vi "Scan For App Projects.vi"(8 "error in":errorcluster, 10 "Init?":bool, 11 "Projects Ref":refnum<vi>) -> (0 "error out":errorcluster)   [LabVIEW 2019, in "Panther Dashboard.lvlib"]
uses:
  Panther Dashboard.lvlib
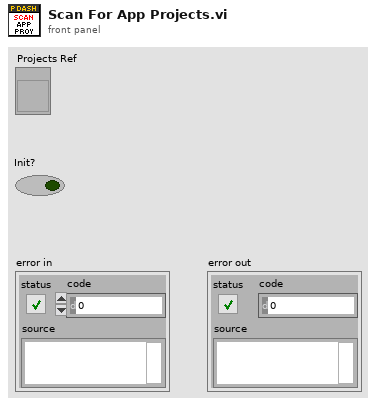
[diagram p1: front panel]
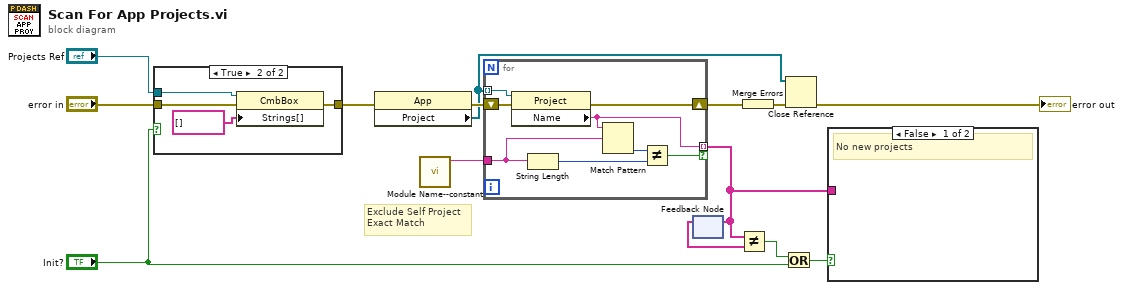
[diagram p0: block diagram]
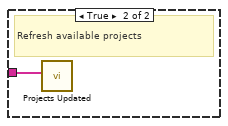
[diagram p3: hidden frame]
diagram:
  # "Exclude Self Project\nExact Match"
  n1 = case shown="True" "Init?" {
    tunnel: "Projects Ref" -> [_ w17]
    tunnel: "error in" -> [w15 w19]
    tunnel: [w15 w18] -> w11
    frame False {
    }
    frame True {
      n2 = property class="CmbBox"(reference=w17, error in=w19, "Strings[]"=string[] []) -> (error out=w18:errorcluster)  [unwired: 1 out]
    }
  }
  n3 = property class="App"(error in=w11) -> (error out=w9:errorcluster, "Project"=w8:refnum<vi>[])  [unwired: 1 in, 1 out]
  n4 = call "Module Name--constant.vi"() -> ("Module Name"=w1:string)  [unwired: 11 in]
  n5 = for {
    tunnel: w8 -> [w22] mode=indexing
    tunnel: [w25] -> w6 mode=indexing if=w23
    tunnel: w1 -> [w21]
    shift-right: [w27] -> w10
    shift-left: w9 -> [w26]
    n6 = property class="Project"(reference=w22, error in=w26) -> (error out=w27:errorcluster, "Name"=w25:string)  [unwired: 1 out]
    n7 = String Length(string=w21) -> (length=w20:i32)
    n8 = Match Pattern(string=w25, regular expression=w21) -> (offset past match=w24:i32)  [unwired: 1 in, 3 out]
    n9 = Not Equal?(x=w24, y=w20) -> (x != y?=w23:bool)
  }
  n10 = feedback-in #1(w6) -> ()
  n11 = feedback #1() -> (w7:string[])  [unwired: 1 in]
  n12 = Not Equal?(x=w6, y=w7) -> (x != y?=w5:bool)
  n13 = Merge Errors(w10) -> (w13:errorcluster)
  n14 = Or(x=w5, y="Init?") -> (x .or. y?=w3:bool)
  n15 = Close Reference(reference=w8, error in (no error)=w13) -> (error out=→"error out":errorcluster)
  n16 = case shown="False" w3 {
    tunnel: w6 -> [_ w28]
    frame False {
      # "No new projects"
    }
    frame True {
      # "Refresh available projects"
      n17 = call "Projects Updated.vi"("Projects"=w28) -> ()  [unwired: 10 in, 1 out]
    }
  }
